vi "Convert Controls to Cluster.vi"(9 "Control Array":string[][](array[string]), 11 "Ctl Properties":T1[](array[typedef])) -> (3 "Ctl Properties out":T1[](array[typedef]))   [LabVIEW 2020, in "VI Properties Editor.lvlib"]
doc: "Converts <B>Control Array</B> and <B>Indicator Array</B> to a cluster array to be used by back-end processes."
uses:
  VI Properties Editor.lvlib
  CTLs/Control Properties.ctl
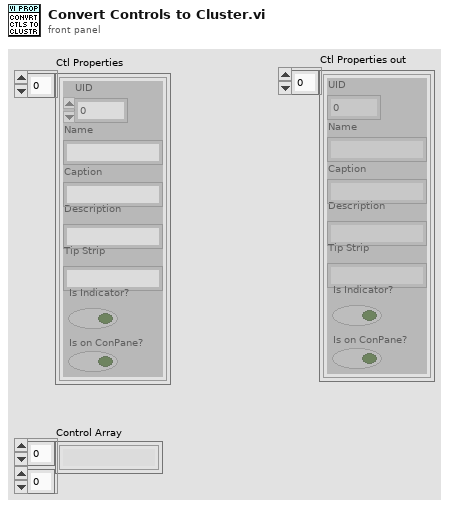
[diagram p1: front panel]
types:
  T1 = typedef "VI Properties Editor.lvlib/Control Properties.ctl" = cluster{"UID":i32, "Name":string, "Caption":string, "Description":string, "Tip Strip":string, "Is Indicator?":bool, "Is on ConPane?":bool}
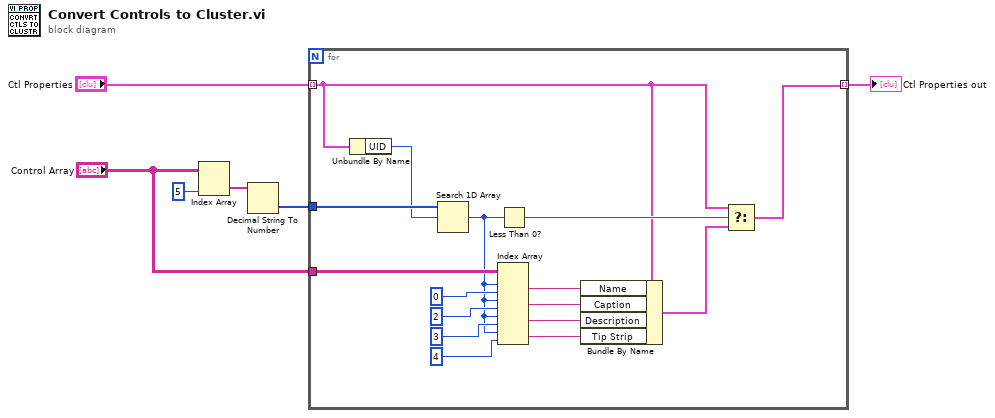
[diagram p0: block diagram]
diagram:
  n1 = Index Array(array="Control Array", index (col)=5 ("disabled index (col)")) -> (element=w3:string[])  [unwired: 1 in]
  n2 = Decimal String To Number(string=w3) -> (number=w2:i32[])  [unwired: 2 in, 1 out]
  n3 = for {
    tunnel: [w10] -> w6 mode=indexing
    tunnel: "Ctl Properties" -> [w12] mode=indexing
    tunnel: w2 -> [w22]
    tunnel: "Control Array" -> [w17]
    n4 = Unbundle By Name(w12) -> ("UID"=w21:i32)
    n5 = Search 1D Array(1D array=w22, element=w21) -> (index of element=w7:i32)  [unwired: 1 in]
    n6 = Index Array(array=w17, index (row) #1=w7, index (col) #1=0 ("disabled index (col)"), index (row) #2=w7, index (col) #2=2 ("disabled index (col)"), index (row) #3=w7, index (col) #3=3 ("disabled index (col)"), index (row) #4=w7, index (col) #4=4 ("disabled index (col)")) -> (element #1=w15:string, element #2=w14:string, element #3=w13:string, element #4=w9:string)
    n7 = Less Than 0?(x=w7) -> (x < 0?=w16:bool)
    n8 = Bundle By Name(cluster=w12, "Name"=w15, "Caption"=w14, "Description"=w13, "Tip Strip"=w9) -> (w11:T1)
    n9 = Select(t=w12, s=w16, f=w11) -> (s? t:f=w10:T1)
  }
  "Ctl Properties out" <- w6
